vi "Timer Demo.vi"   [LabVIEW 2020]
uses:
  Timer Demo App/Timer Demo App.lvclass
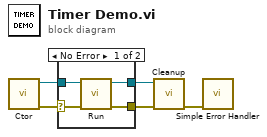
[diagram p0: block diagram]
diagram:
  n1 = call "Ctor.vi"() -> ("error out"=w5:errorcluster, "Timer Demo App out"=w4:refnum<class "Timer Demo App.lvclass">)  [unwired: 10 in]
  n2 = case shown="No Error" w5 {
    selector: w5 -> [w8 w10]
    tunnel: w4 -> [w9 w11]
    tunnel: [w7 w10] -> w2
    tunnel: [w6 w11] -> w3
    frame No Error {
      n3 = call "Run.vi"("error in (no error)"=w8, "Timer Demo App in"=w9) -> ("error out"=w7:errorcluster, "Timer Demo App out"=w6:refnum<class "Timer Demo App.lvclass">)  [unwired: 8 in]
    }
    frame Error {
    }
  }
  n4 = call "Cleanup.vi"("error in (no error)"=w2, "Timer Demo App in"=w3) -> ("error out"=w1:errorcluster)  [unwired: 9 in]
  n5 = call <vilib>:"Simple Error Handler.vi"("error in (no error)"=w1) -> ()  [unwired: 4 in, 5 out]
